vi "Advent of Code 2022 Day 1.vi"() -> ()   [LabVIEW 2020]
panel:
  out "Step Two Answer":i32
  out "Step One Answer":i32
  in  "Input String":string
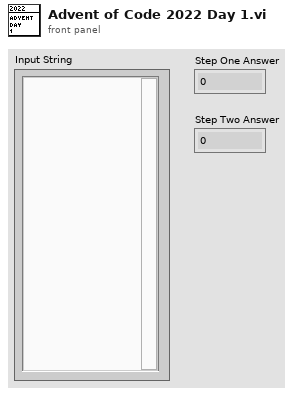
[diagram p1: front panel]
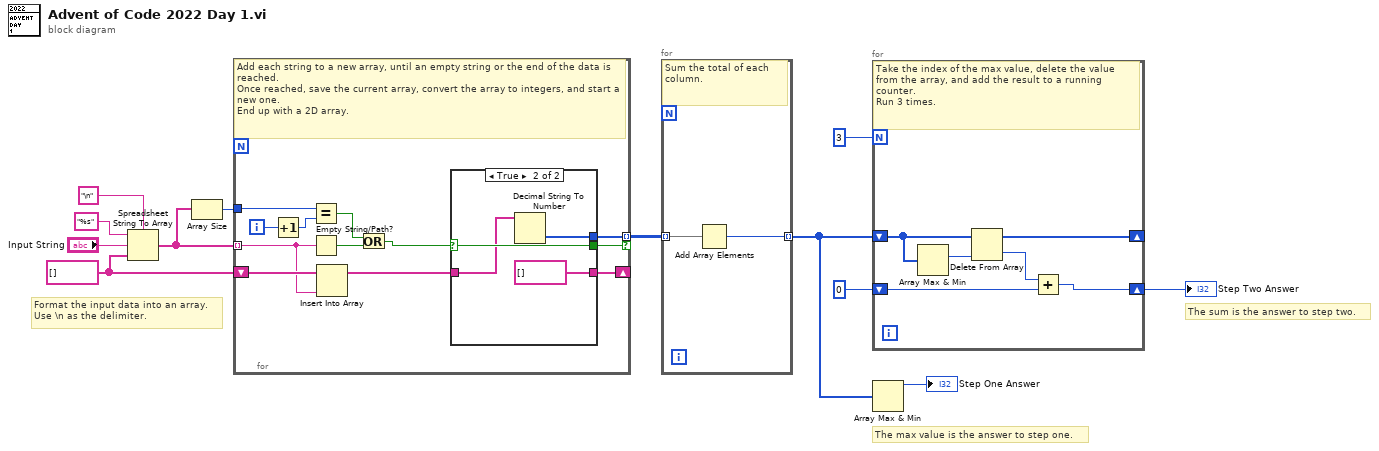
[diagram p0: block diagram]
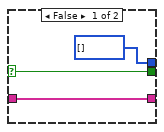
[diagram p2: hidden frame]
diagram:
  w9 = string[] []
  # "The sum is the answer to step two."
  # "The max value is the answer to step one."
  # "Format the input data into an array.\nUse \\n as the delimiter."
  n1 = Spreadsheet String To Array(delimiter (Tab)="\n", format string="%s", spreadsheet string="Input String", array type (2D Dbl)=w9) -> (array=w3:string[])
  n2 = Array Size(array=w3) -> (size(s)=w2:i32)
  n3 = for {
    tunnel: w3 -> [w23] mode=indexing
    shift-right: [w21] -> _
    shift-left: w9 -> [w24]
    tunnel: [w19] -> w1 mode=indexing if=w20
    tunnel: w2 -> [w18]
    i -> [w14]
    # "Add each string to a new array, until an empty string or the end of the data is reached.\nOnce reached, save the current array, convert the array to integers, and start a new one.\nEnd up with a 2D array."
    n4 = Increment(x=w14) -> (x+1=w13:i32)
    n5 = Equal?(x=w18, y=w13) -> (x = y?=w16:bool)
    n6 = Empty String/Path?(string/path=w23) -> (empty?=w17:bool)
    n7 = Insert Into Array(array=w24, new element=w23) -> (w22:string[])  [unwired: 1 in]
    n8 = Or(x=w16, y=w17) -> (x .or. y?=w15:bool)
    n9 = case shown="True" w15 {
      selector: w15 -> [w27 w30]
      tunnel: w22 -> [w26 w29]
      tunnel: [w26 string[] []] -> w21
      tunnel: [w27 w30] -> w20
      tunnel: [i32[] [] w28] -> w19
      frame False {
      }
      frame True {
        n10 = Decimal String To Number(string=w29) -> (number=w28:i32[])  [unwired: 2 in, 1 out]
      }
    }
  }
  n11 = for {
    tunnel: w1 -> [w33] mode=indexing
    tunnel: [w32] -> w7 mode=indexing
    # "Sum the total of each column."
    n12 = Add Array Elements(numeric array=w33) -> (sum=w32:i32)
  }
  n13 = for {
    N: 3 -> [_]
    shift-right: [w37] -> _
    shift-left: w7 -> [w39]
    shift-right: [w36] -> w4
    shift-left: 0 -> [w35]
    # "Take the index of the max value, delete the value from the array, and add the result to a running counter.\nRun 3 times."
    n14 = Array Max & Min(array=w39) -> (max index (indices)=w38:i32)  [unwired: 3 out]
    n15 = Delete From Array(array=w39, index=w38) -> (deleted portion=w34:i32, array with subset deleted=w37:i32[])  [unwired: 1 in]
    n16 = Add(x=w34, y=w35) -> (x+y=w36:i32)
  }
  "Step Two Answer" <- w4
  n17 = Array Max & Min(array=w7) -> (max value=→"Step One Answer":i32)  [unwired: 3 out]
